vi "Text Description.vi"(11 "Message":refnum<class "Observer_RegisterForAll.lvclass">) -> (2 "Description":string, 3 "Message":refnum<class "Observer_RegisterForAll.lvclass">)   [LabVIEW 2011, in "Messenging.lvlib" / "Observer_RegisterForAll.lvclass"]
uses:
  Observer_RegisterForAll.lvclass
  ParentCommand/ObserverRegistryCommand.lvclass
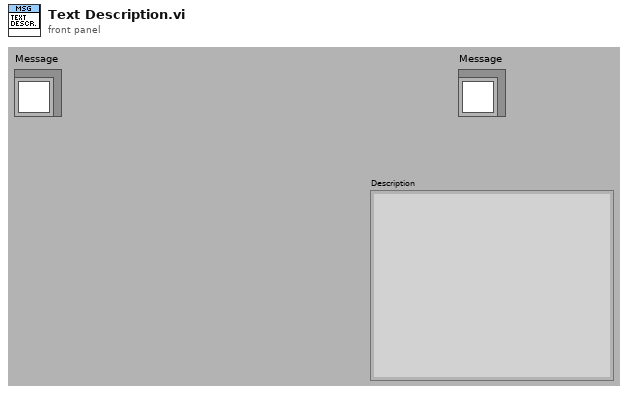
[diagram p1: front panel]
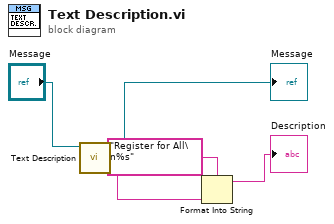
[diagram p0: block diagram]
diagram:
  n1 = call-parent "Text Description.vi"("Message"="Message") -> ("Description"=w3:string, "Message"=→"Message":refnum<class "Observer_RegisterForAll.lvclass">)  [unwired: 9 out]
  n2 = Format Into String(format string="Register for All\n%s", w3) -> (resulting string=→"Description":string)  [unwired: 2 in, 1 out]
